vi "S2C_ExeScriptResume.vi"(8 "Error In":errorcluster, 11 "Q-Ref":refnum<queue>) -> (0 "Error Out":errorcluster)   [LabVIEW 2015]
doc: "Calls the run case, causing the execution to continue."
uses:
  Globals/S2C_Globals.vi
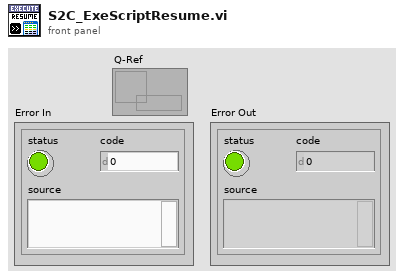
[diagram p1: front panel]
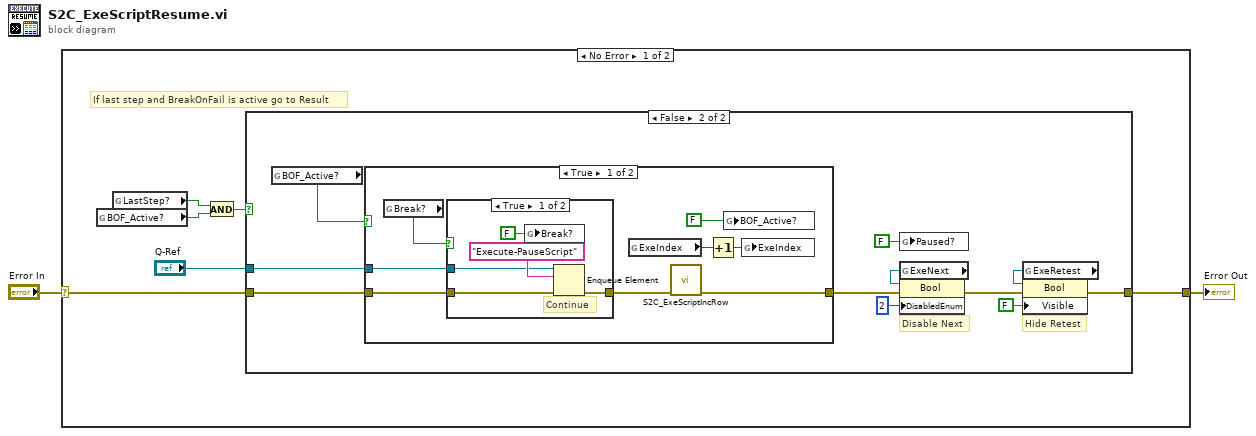
[diagram p0: block diagram]
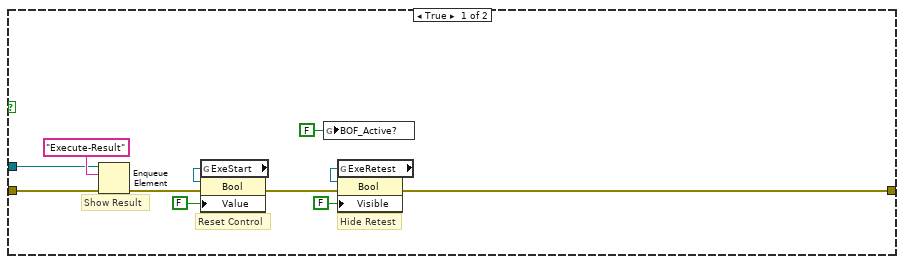
[diagram p2: hidden frame]
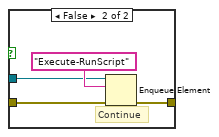
[diagram p3: hidden frame]
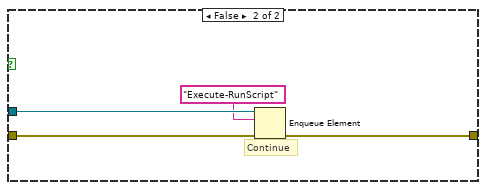
[diagram p4: hidden frame]
diagram:
  n1 = case shown="No Error" "Error In" {
    selector: "Error In" -> [w7 w52]
    tunnel: [w6 w52] -> w1
    frame No Error {
      # "If last step and BreakOnFail is active go to Result"
      n2 = global read "S2C_Globals.vi" "BOF_Active?"() -> (w5:bool)
      n3 = global read "S2C_Globals.vi" "LastStep?"() -> (w4:bool)
      n4 = And(x=w4, y=w5) -> (x .and. y?=w3:bool)
      n5 = case shown="False" w3 {
        tunnel: "Q-Ref" -> [w10 w20]
        tunnel: w7 -> [w11 w23]
        tunnel: [w9 w21] -> w6
        frame True {
          # "Hide Retest"
          # "Show Result"
          # "Reset Control"
          n6 = Enqueue Element(queue=w10, element="Execute-Result", error in (no error)=w11) -> (error out=w13:errorcluster)  [unwired: 1 in, 2 out]
          n7 = global read "S2C_Globals.vi" "ExeStart"() -> (w15:refnum<vi>)
          n8 = property class="Bool"(reference=w15, error in=w13, "Value"=FALSE) -> (error out=w18:errorcluster)  [unwired: 1 out]
          n9 = global write "S2C_Globals.vi" "BOF_Active?"(FALSE ("BOF_Active?")) -> ()
          n10 = global read "S2C_Globals.vi" "ExeRetest"() -> (w16:refnum<vi>)
          n11 = property on="Property Node" class="Bool"(reference=w16, error in=w18, "Visible"=FALSE) -> (error out=w9:errorcluster)  [unwired: 1 out]
        }
        frame False {
          # "Hide Retest"
          # "Disable Next"
          n12 = global read "S2C_Globals.vi" "BOF_Active?"() -> (w24:bool)
          n13 = case shown="True" w24 {
            tunnel: w23 -> [w34 w51]
            tunnel: [w35 w49] -> w22
            tunnel: w20 -> [w31 w50]
            frame True {
              n14 = global read "S2C_Globals.vi" "Break?"() -> (w32:bool)
              n15 = case shown="True" w32 {
                tunnel: w34 -> [w42 w46]
                tunnel: [w41 w45] -> w33
                tunnel: w31 -> [w39 w44]
                frame True {
                  # "Continue"
                  n16 = global write "S2C_Globals.vi" "Break?"(FALSE ("Break?")) -> ()
                  n17 = Enqueue Element(queue=w39, element="Execute-PauseScript", error in (no error)=w42) -> (error out=w41:errorcluster)  [unwired: 1 in, 2 out]
                }
                frame False {
                  # "Continue"
                  n18 = Enqueue Element(queue=w44, element="Execute-RunScript", error in (no error)=w46) -> (error out=w45:errorcluster)  [unwired: 1 in, 2 out]
                }
              }
              n19 = global read "S2C_Globals.vi" "ExeIndex"() -> (w37:i32)
              n20 = call "S2C_ExeScriptIncRow.vi"("Error In"=w33) -> ("Error Out"=w35:errorcluster)  [unwired: 10 in]
              n21 = Increment(x=w37) -> (x+1=w36:i32)
              n22 = global write "S2C_Globals.vi" "BOF_Active?"(FALSE ("BOF_Active?")) -> ()
              n23 = global write "S2C_Globals.vi" "ExeIndex"(w36) -> ()
            }
            frame False {
              # "Continue"
              n24 = Enqueue Element(queue=w50, element="Execute-RunScript", error in (no error)=w51) -> (error out=w49:errorcluster)  [unwired: 1 in, 2 out]
            }
          }
          n25 = global write "S2C_Globals.vi" "Paused?"(FALSE ("Paused?")) -> ()
          n26 = global read "S2C_Globals.vi" "ExeNext"() -> (w30:refnum<vi>)
          n27 = property on="Property Node" class="Bool"(reference=w30, error in=w22, "DisabledEnum"=u8 2) -> (error out=w26:errorcluster)  [unwired: 1 out]
          n28 = global read "S2C_Globals.vi" "ExeRetest"() -> (w27:refnum<vi>)
          n29 = property on="Property Node" class="Bool"(reference=w27, error in=w26, "Visible"=FALSE) -> (error out=w21:errorcluster)  [unwired: 1 out]
        }
      }
    }
    frame Error {
    }
  }
  "Error Out" <- w1
